vi "SelectOPCTags.RecurseThroughOPCTags.vi"(6 "LUT":variant, 8 "error in (no error)":errorcluster, 9 "Parent Tag":string, 10 "reference out":refnum<vi>, 11 "OPC UA Client Ref":refnum<k21>) -> (0 "error out":errorcluster, 3 "OPC UA Client Ref":refnum<k21>, 4 "LUT":variant)   [LabVIEW 2015, in "OPC UA Client System Explorer.lvlib"]
uses:
  OPC UA Client System Explorer.lvlib
  Types/Tag.TreeSettings.ctl
  SelectOPCTags.GetNodeAttribute.vi
  <vilib>/OPCUA/client/Read.vi
  <vilib>/OPCUA/client/Read ByteString.vi
  <vilib>/OPCUA/client/Read Double Array.vi
  <vilib>/OPCUA/client/Read Float Array.vi
  <vilib>/OPCUA/client/Read UInt32 Array.vi
  <vilib>/OPCUA/client/Read Int32 Array.vi
  <vilib>/OPCUA/client/Read UInt16 Array.vi
  <vilib>/OPCUA/client/Read Int16 Array.vi
  <vilib>/OPCUA/client/Read Byte Array.vi
  <vilib>/OPCUA/client/Read SByte Array.vi
  <vilib>/OPCUA/client/Read Bool Array.vi
  <vilib>/OPCUA/client/Read UInt64 Array.vi
  <vilib>/OPCUA/client/Read Int64 Array.vi
  <vilib>/OPCUA/client/Read DateTime Array.vi
  <vilib>/OPCUA/NI OPC UA Client.lvlib
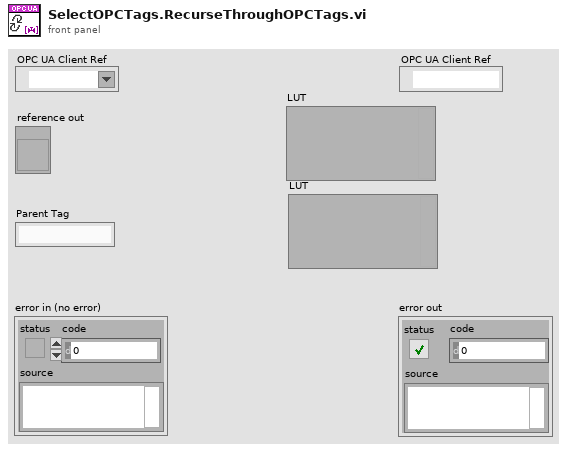
[diagram p1: front panel]
types:
  T1 = cluster{"node path":string, "node name":string, "node type":enum32{"Other", "Folder", "Item/Property"}}[]
  T2 = typedef "OPC UA Client System Explorer.lvlib/Tag.TreeSettings.ctl" = cluster{"Settings":cluster{"name":string, "node type":enum32{"Other", "Folder", "Item/Property"}, "DataType":u32, "access":enum16{"Null", "Read", "Write", "Read&Write"}, "description":string}, "Array Size":i32}
  T3 = cluster{"name":string, "node type":enum32{"Other", "Folder", "Item/Property"}, "DataType":u32, "access":enum16{"Null", "Read", "Write", "Read&Write"}, "description":string}
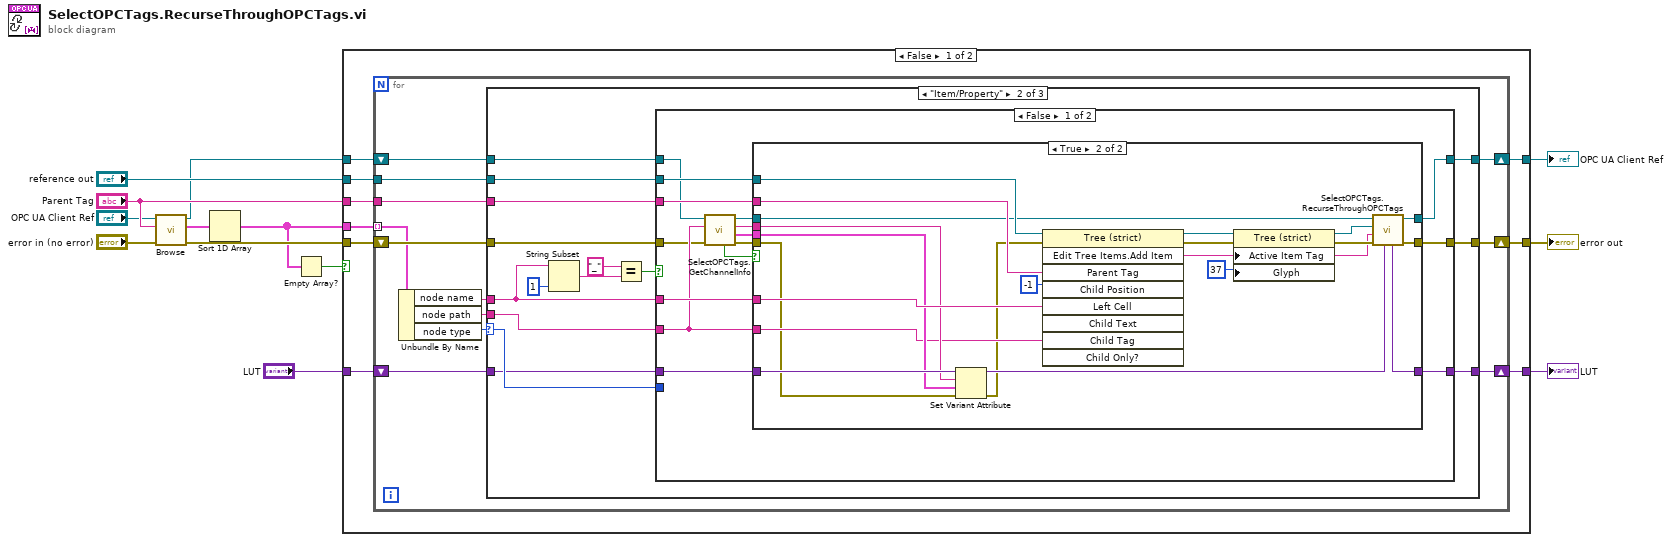
[diagram p0: block diagram]
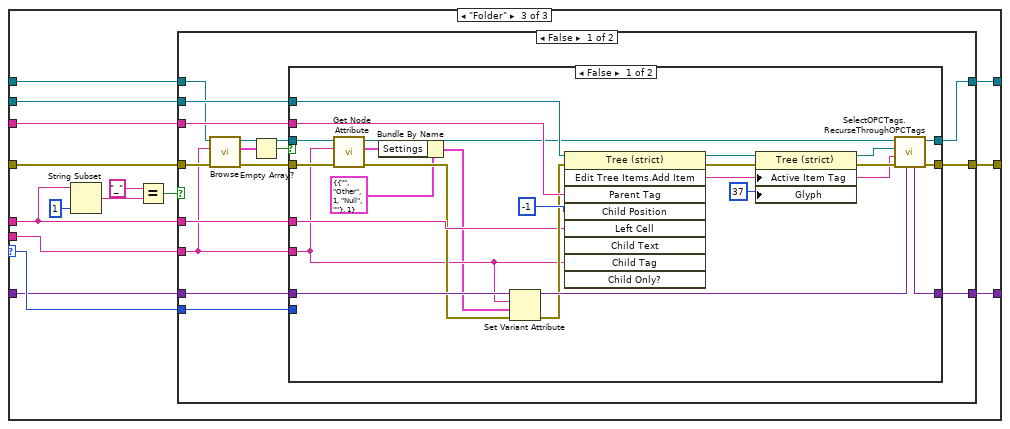
[diagram p5: hidden frame]
diagram:
  n1 = call <vilib>:"Browse.vi"("error in (no error)"="error in (no error)", "node path"="Parent Tag", "OPC UA client refnum in"="OPC UA Client Ref") -> ("error out"=w13:errorcluster, "browse result"=w11:T1, "OPC UA client refnum out"=w5:refnum<k21>)  [unwired: 5 in, 1 out]
  n2 = Sort 1D Array(array=w11) -> (sorted array=w1:T1)
  n3 = Empty Array?(array=w1) -> (empty?=w10:bool)
  n4 = case shown="False" w10 {
    tunnel: w13 -> [w22 w157]
    tunnel: "reference out" -> [w21 _]
    tunnel: [w20 w157] -> w7
    tunnel: "Parent Tag" -> [w19 _]
    tunnel: w1 -> [w18 _]
    tunnel: w5 -> [w17 w156]
    tunnel: [w16 w156] -> w4
    tunnel: [w15 w155] -> w3
    tunnel: "LUT" -> [w14 w155]
    frame False {
      n5 = for {
        tunnel: w18 -> [w33] mode=indexing
        tunnel: w19 -> [w29]
        shift-right: [w28] -> w20
        shift-left: w22 -> [w34]
        tunnel: w21 -> [w30]
        shift-right: [w26] -> w16
        shift-left: w17 -> [w27]
        shift-right: [w24] -> w15
        shift-left: w14 -> [w23]
        n6 = Unbundle By Name(w33) -> ("node name"=w32:string, "node path"=w31:string, "node type"=w25:enum32{"Other", "Folder", "Item/Property"})
        n7 = case shown="\"Item/Property\"" w25 {
          selector: w25 -> [_ w40 w97]
          tunnel: w34 -> [w37 w52 w109]
          tunnel: w32 -> [_ w45 w102]
          tunnel: w31 -> [_ w51 w108]
          tunnel: w30 -> [_ w50 w107]
          tunnel: w29 -> [_ w49 w106]
          tunnel: [w37 w48 w105] -> w28
          tunnel: w27 -> [w36 w47 w104]
          tunnel: [w36 w46 w103] -> w26
          tunnel: [w35 w39 w96] -> w24
          tunnel: w23 -> [w35 w38 w95]
          frame "Other" {
          }
          frame "Item/Property" {
            n8 = String Subset(string=w45, length (rest)=1 ("length (rest)")) -> (substring=w43:string)  [unwired: 1 in]
            n9 = Equal?(x="_", y=w43) -> (x = y?=w41:bool)
            n10 = case shown="False" w41 {
              tunnel: w52 -> [w54 w94]
              tunnel: w51 -> [w56 _]
              tunnel: w50 -> [w67 _]
              tunnel: w49 -> [w66 _]
              tunnel: [w65 w94] -> w48
              tunnel: w47 -> [w60 w93]
              tunnel: [w64 w93] -> w46
              tunnel: w45 -> [w63 _]
              tunnel: w40 -> [_ _]
              tunnel: [w61 w92] -> w39
              tunnel: w38 -> [w62 w92]
              frame False {
                n11 = call "SelectOPCTags.GetChannelInfo.vi"("error in (no error)"=w54, "Item URL"=w56, "OPC UA client refnum in"=w60) -> ("error out"=w55:errorcluster, "Setings"=w58:T2, "Item URL out"=w57:string, "OPC UA client refnum out"=w59:refnum<k21>, "Use"=w53:bool)  [unwired: 4 in]
                n12 = case shown="True" w53 {
                  tunnel: w67 -> [_ w91]
                  tunnel: w66 -> [_ w90]
                  tunnel: [w70 w89] -> w65
                  tunnel: [w68 w88] -> w64
                  tunnel: w63 -> [_ w87]
                  tunnel: w62 -> [w69 w82]
                  tunnel: [w69 w80] -> w61
                  tunnel: w59 -> [w68 w78]
                  tunnel: w58 -> [_ w77]
                  tunnel: w57 -> [_ w76]
                  tunnel: w56 -> [_ w74]
                  tunnel: w55 -> [w70 w72]
                  frame False {
                  }
                  frame True {
                    n13 = Set Variant Attribute(Variant=w82, name=w76, value=w77, error in=w72) -> (Variant out=w81:variant, error out=w71:errorcluster)  [unwired: 1 out]
                    n14 = invoke class="Tree (strict)" method="Edit Tree Items.Add Item"(reference=w91, error in=w71, "Parent Tag"=w90, "Child Position"=-1, "Left Cell"=w87, "Child Tag"=w74) -> (reference out=w85:refnum<vi>, error out=w86:errorcluster, "Edit Tree Items:Add Item"=w73:string)  [unwired: 3 in, 6 out]
                    n15 = property class="Tree (strict)"(reference=w85, error in=w86, "Active Item Tag"=w73, "Glyph"=37 ("Active Item:Symbol Index")) -> (reference out=w84:refnum<vi>, error out=w75:errorcluster)
                    n16 = call "SelectOPCTags.RecurseThroughOPCTags.vi"("LUT"=w81, "error in (no error)"=w75, "Parent Tag"=w73, "reference out"=w84, "OPC UA Client Ref"=w78) -> ("error out"=w89:errorcluster, "OPC UA Client Ref"=w88:refnum<k21>, "LUT"=w80:variant)  [unwired: 4 in]
                  }
                }
              }
              frame True {
              }
            }
          }
          frame "Folder" {
            n17 = String Subset(string=w102, length (rest)=1 ("length (rest)")) -> (substring=w100:string)  [unwired: 1 in]
            n18 = Equal?(x="_", y=w100) -> (x = y?=w98:bool)
            n19 = case shown="False" w98 {
              tunnel: w109 -> [w116 w154]
              tunnel: w108 -> [w110 _]
              tunnel: w107 -> [w124 _]
              tunnel: w106 -> [w123 _]
              tunnel: [w122 w154] -> w105
              tunnel: w104 -> [w114 w153]
              tunnel: [w121 w153] -> w103
              tunnel: w102 -> [w120 _]
              tunnel: w97 -> [w111 _]
              tunnel: [w118 w152] -> w96
              tunnel: w95 -> [w119 w152]
              frame False {
                n20 = call <vilib>:"Browse.vi"("error in (no error)"=w116, "node path"=w110, "OPC UA client refnum in"=w114) -> ("error out"=w115:errorcluster, "browse result"=w117:T1, "OPC UA client refnum out"=w113:refnum<k21>)  [unwired: 5 in, 1 out]
                n21 = Empty Array?(array=w117) -> (empty?=w112:bool)
                n22 = case shown="False" w112 {
                  tunnel: w124 -> [w148 _]
                  tunnel: w123 -> [w147 _]
                  tunnel: [w146 w150] -> w122
                  tunnel: [w145 w151] -> w121
                  tunnel: w120 -> [w133 _]
                  tunnel: w119 -> [w144 w149]
                  tunnel: [w143 w149] -> w118
                  tunnel: w110 -> [w128 _]
                  tunnel: w115 -> [w132 w150]
                  tunnel: w113 -> [w130 w151]
                  tunnel: w111 -> [_ _]
                  frame False {
                    n23 = call <vilib>:"Get Node Attribute.vi"("error in (no error)"=w132, "node path"=w128, "OPC UA client refnum in"=w130) -> ("error out"=w131:errorcluster, "node attribute"=w126:T3, "OPC UA client refnum out"=w129:refnum<k21>)  [unwired: 6 in]
                    n24 = Bundle By Name(cluster=T2 {"Settings"={"name"="", "node type"=enum."Other", "DataType"=1, "access"=enum."Null", "description"=""}, "Array Size"=1}, "Settings"=w126) -> (w125:T2)
                    n25 = Set Variant Attribute(Variant=w144, name=w128, value=w125, error in=w131) -> (Variant out=w138:variant, error out=w134:errorcluster)  [unwired: 1 out]
                    n26 = invoke class="Tree (strict)" method="Edit Tree Items.Add Item"(reference=w148, error in=w134, "Parent Tag"=w147, "Child Position"=-1, "Left Cell"=w133, "Child Tag"=w128) -> (reference out=w141:refnum<vi>, error out=w142:errorcluster, "Edit Tree Items:Add Item"=w135:string)  [unwired: 3 in, 6 out]
                    n27 = property class="Tree (strict)"(reference=w141, error in=w142, "Active Item Tag"=w135, "Glyph"=37 ("Active Item:Symbol Index")) -> (reference out=w140:refnum<vi>, error out=w136:errorcluster)
                    n28 = call "SelectOPCTags.RecurseThroughOPCTags.vi"("LUT"=w138, "error in (no error)"=w136, "Parent Tag"=w135, "reference out"=w140, "OPC UA Client Ref"=w129) -> ("error out"=w146:errorcluster, "OPC UA Client Ref"=w145:refnum<k21>, "LUT"=w143:variant)  [unwired: 4 in]
                  }
                  frame True {
                  }
                }
              }
              frame True {
              }
            }
          }
        }
      }
    }
    frame True {
    }
  }
  "OPC UA Client Ref" <- w4
  "error out" <- w7
  "LUT" <- w3
